vi "arydh -- get one readings.vi"(7 "channelicicle":T1, 11 "MCL object":T4) -> (2 "reading":cdb, 3 "MCL object OUT":T4)   [LabVIEW 2018]
uses:
  nanocal/Nanocalorimetry/data/MCL.lvlibp/MCL library/MCL_DataRef.ctl
  channelicicle.ctl
  nanocal/Nanocalorimetry/data/MCL.lvlibp/SynkTek FPGA/FPGA_SharedResources/FPGASharedResources_Readings_ReadingChannelTypedef.ctl
  nanocal/Nanocalorimetry/data/MCL.lvlibp/SynkTek FPGA/FPGA_SharedResources/FPGASharedResources_Lockin_Typedef.ctl
  nanocal/Nanocalorimetry/data/MCL.lvlibp/SynkTek FPGA/FPGA_SharedResources/FPGASharedResources_PhaseType_Typedef.ctl
  nanocal/Nanocalorimetry/data/MCL.lvlibp
  nanocal/Nanocalorimetry/data/MCL.lvlibp/SynkTek FPGA/FPGA_SharedResources/FPGA_SharedResources.lvlib
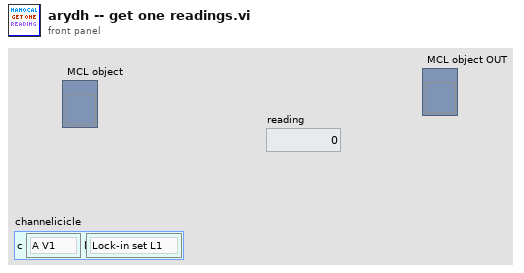
[diagram p1: front panel]
types:
  T1 = typedef "channelicicle.ctl" = cluster{"c":T2, "l":T3}
  T2 = typedef "MCL.lvlibp/FPGA_SharedResources.lvlib/FPGASharedResources_Readings_ReadingChannelTypedef.ctl" = enum8{"A V1", "A V2", "B V1", "B V2", "C V1", "C V2", "D V1", "D V2", "E V1", "E V2", "A I", "B I", "C I", "D I", "E I", "Int."}
  T3 = typedef "MCL.lvlibp/FPGA_SharedResources.lvlib/FPGASharedResources_Lockin_Typedef.ctl" = enum8{"Lock-in set L1", "Lock-in set L2"}
  T4 = typedef "MCL.lvlibp/MCL_DataRef.ctl" = refnum<vi>
  T5 = typedef "MCL.lvlibp/FPGA_SharedResources.lvlib/FPGASharedResources_PhaseType_Typedef.ctl" = enum16{"DC", "X", "Y", "R", "Theta"}
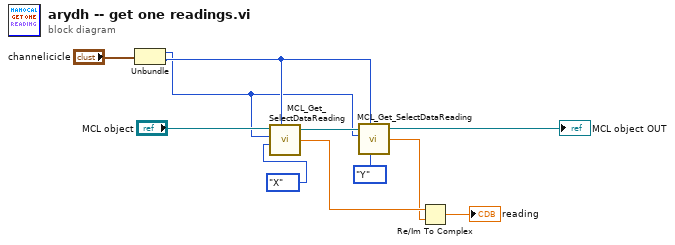
[diagram p0: block diagram]
diagram:
  n1 = Unbundle("channelicicle") -> ("c"=w1:T2, "l"=w2:T3)
  n2 = call "MCL_Get_SelectDataReading.vi"("MCL object"="MCL object", "Reading Ch"=w1, "PhaseType"=FPGASharedResources_PhaseType_Typedef."X", "Lockin"=w2) -> ("MCL object"=w9:T4, "Select reading"=w7:dbl)  [unwired: 1 in, 1 out]
  n3 = call "MCL_Get_SelectDataReading.vi"("MCL object"=w9, "Reading Ch"=w1, "PhaseType"=FPGASharedResources_PhaseType_Typedef."Y", "Lockin"=w2) -> ("MCL object"=→"MCL object OUT":T4, "Select reading"=w6:dbl)  [unwired: 1 in, 1 out]
  n4 = Re/Im To Complex(1:w6, 2:w7) -> (0:→"reading":cdb)
